vi "SLG_ArrayToString_Array.vi"(1 "OrArray":string[](array[string]), 3 "SLG_Array":sgl[](array[numeric])) -> (0 "StringArray":string[](array[string]))   [LabVIEW 2019]
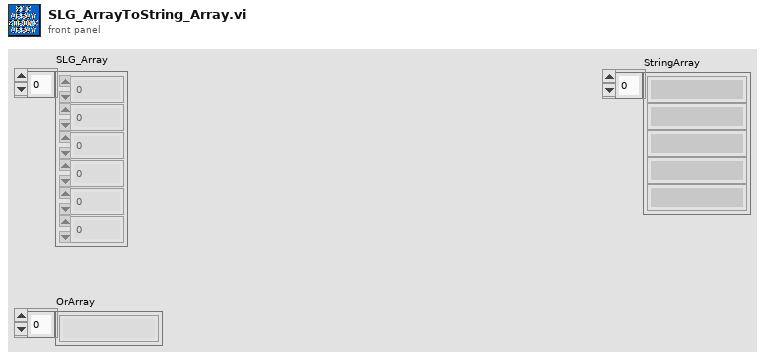
[diagram p1: front panel]
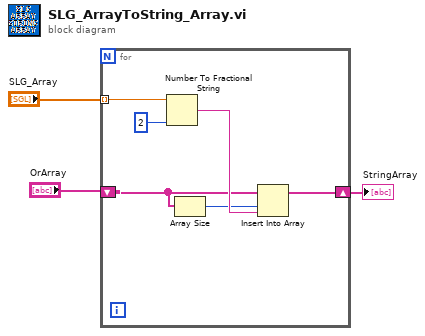
[diagram p0: block diagram]
diagram:
  n1 = for {
    tunnel: "SLG_Array" -> [w8] mode=indexing
    shift-right: [w9] -> w2
    shift-left: "OrArray" -> [w6]
    n2 = Number To Fractional String(number=w8, precision (6)=2) -> (F-format string=w7:string)  [unwired: 2 in]
    n3 = Array Size(array=w6) -> (size(s)=w5:i32)
    n4 = Insert Into Array(array=w6, index=w5, new element=w7) -> (w9:string[])
  }
  "StringArray" <- w2
